vi "Online Judge Repair.vi"(8 "error in (no error)":errorcluster caption="错误输入（无错误）", 10 "Online_Table":T1, 11 "conn refer":T2) -> (0 "error out":errorcluster, 2 "Steps":string[](array[string]), 3 "Online_Table out":T1)   [LabVIEW 2014]
uses:
  Type'def/Online_Table.ctl
  <vilib>/addons/database/_DB Variant To Data/Database Variant To Data.xnode
  Database/Ctr/Constr.ctl
  <vilib>/addons/database/Connection.llb/Conn ObjectReference.ctl
  <vilib>/addons/database/NI_Database_API.lvlib
  Database/Ctr/Conneect State.ctl
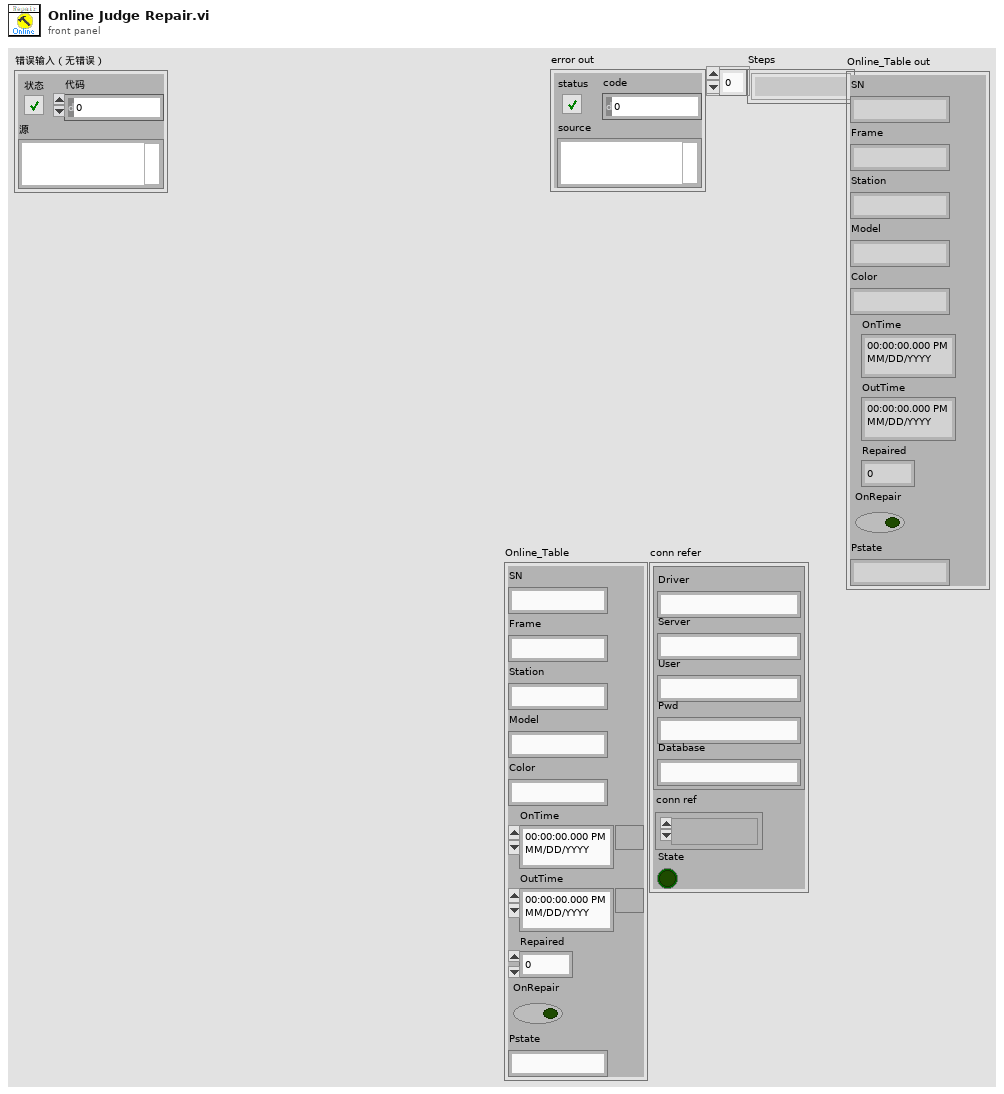
[diagram p1: front panel]
types:
  T1 = typedef "Online_Table.ctl" = cluster{"SN":string, "Frame":string, "Station":string, "Model":string, "Color":string, "OnTime":timestamp, "OutTime":timestamp, "Repaired":i32, "OnRepair":bool, "Pstate":string}
  T2 = typedef "Conneect State.ctl" = cluster{"Constr":T3, "conn ref":T4, "State":bool}
  T3 = typedef "Constr.ctl" = cluster{"Driver":string, "Server":string, "User":string, "Pwd":string, "Database":string}
  T4 = typedef "NI_Database_API.lvlib/Conn ObjectReference.ctl" = refnum<k1>
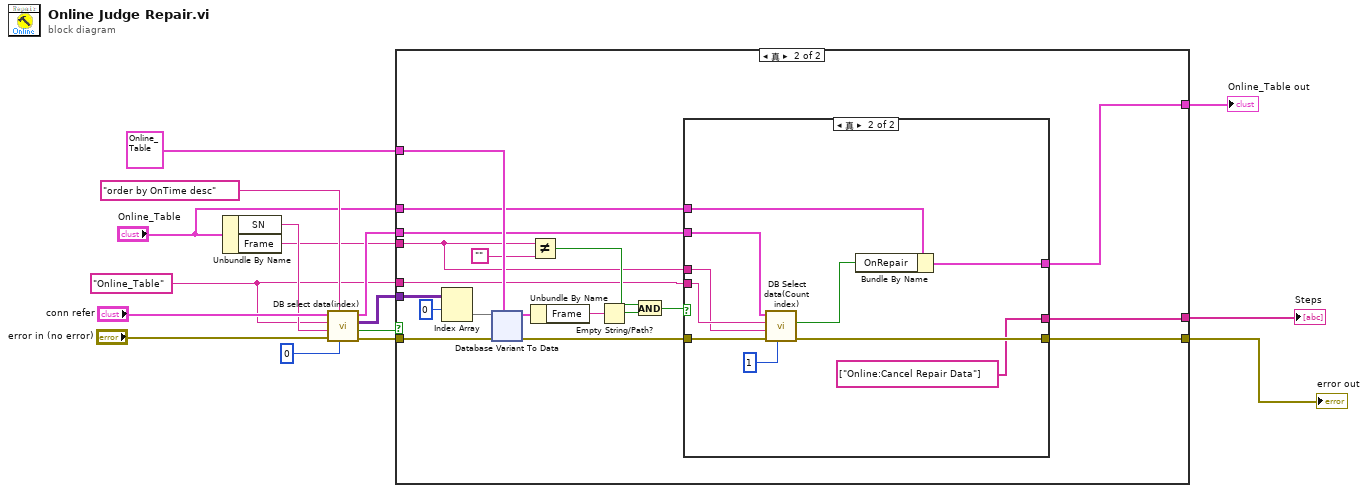
[diagram p0: block diagram]
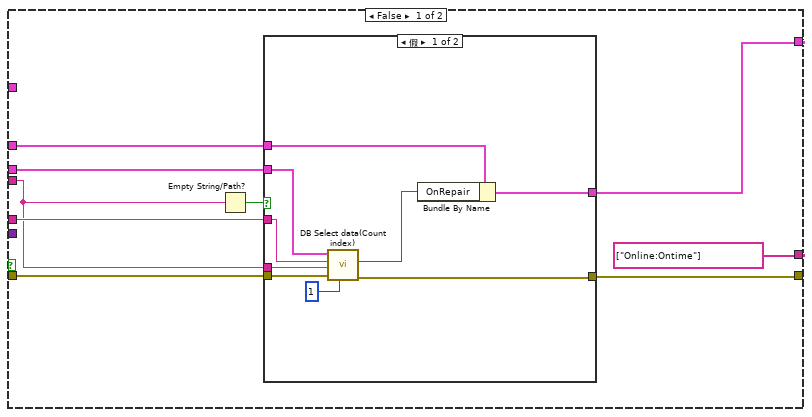
[diagram p2: hidden frame]
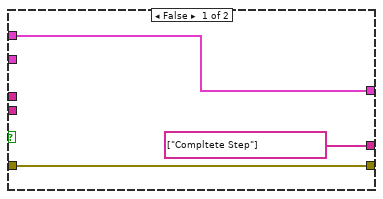
[diagram p4: hidden frame]
diagram:
  w6 = "Online_Table" ("Tabe")
  n1 = Unbundle By Name("Online_Table") -> ("SN"=w14:string, "Frame"=w4:string)
  n2 = call "DB select data(index).vi"("index"=0, "Condtion"="order by OnTime desc", "error in (no error)"="error in (no error)", "Code"=w14, "Tabe"=w6, "Connncet State"="conn refer") -> ("error out"=w12:errorcluster, "state"=w11:bool, "data"=w8:variant[][], "Connncet State out"=w7:T2)  [unwired: 2 in]
  n3 = case shown="真" w11 {
    tunnel: w12 -> [w18 w53]
    tunnel: T1 {"SN"="", "Frame"="", "Station"="", "Model"="", "Color"="", "OnTime"=timestamp(0 s since 1904-01-01), "OutTime"=timestamp(0 s since 1904-01-01), "Repaired"=0, "OnRepair"=FALSE, "Pstate"=""} ("Online_Table") -> [_ w52]
    tunnel: w8 -> [_ w55]
    tunnel: w7 -> [w24 w42]
    tunnel: w6 -> [w23 w41]
    tunnel: "Online_Table" -> [w22 w43]
    tunnel: [w21 w39] -> w1
    tunnel: [string[] ["Online:Ontime"] w37] -> w2
    tunnel: w4 -> [w19 w40]
    tunnel: [w17 w38] -> w3
    frame False {
      n4 = Empty String/Path?(string/path=w19) -> (empty?=w25:bool)
      n5 = case shown="假" w25 {
        tunnel: w18 -> [w34 w36]
        tunnel: w24 -> [w33 _]
        tunnel: w19 -> [w31 _]
        tunnel: w23 -> [w32 _]
        tunnel: w22 -> [w29 w35]
        tunnel: [w27 w36] -> w17
        tunnel: [w26 w35] -> w21
        frame False {
          n6 = call "DB Select data(Count index).vi"("index"=1, "error in (no error)"=w34, "Code"=w31, "Tabe"=w32, "Connncet State"=w33) -> ("error out"=w27:errorcluster, "state"=w28:bool)  [unwired: 3 in, 2 out]
          n7 = Bundle By Name(cluster=w29, "OnRepair"=w28) -> (w26:T1)
        }
        frame True {
        }
      }
    }
    frame True {
      n8 = Index Array(array=w55, index (row)=0) -> (element=w51:variant[])  [unwired: 1 in]
      n9 = xnode "Database Variant To Data"("database variant"=w51, "error in (no error)"=w53, "type"=w52) -> ("data"=w50:T1, "error out"=w44:errorcluster)
      n10 = Not Equal?(x=w40, y="") -> (x != y?=w46:bool)
      n11 = Unbundle By Name(w50) -> ("Frame"=w48:string)
      n12 = Empty String/Path?(string/path=w48) -> (empty?=w47:bool)
      n13 = And(x=w46, y=w47) -> (x .and. y?=w45:bool)
      n14 = case shown="真" w45 {
        tunnel: w44 -> [w57 w66]
        tunnel: w43 -> [w58 w65]
        tunnel: w42 -> [_ w64]
        tunnel: w41 -> [_ w63]
        tunnel: w40 -> [_ w62]
        tunnel: [w58 w61] -> w39
        tunnel: [w57 w60] -> w38
        tunnel: [string[] ["Compltete Step"] string[] ["Online:Cancel Repair Data"]] -> w37
        frame False {
        }
        frame True {
          n15 = call "DB Select data(Count index).vi"("index"=1, "error in (no error)"=w66, "Code"=w62, "Tabe"=w63, "Connncet State"=w64) -> ("error out"=w60:errorcluster, "state"=w67:bool)  [unwired: 3 in, 2 out]
          n16 = Bundle By Name(cluster=w65, "OnRepair"=w67) -> (w61:T1)
        }
      }
    }
  }
  "error out" <- w3
  "Steps" <- w2
  "Online_Table out" <- w1
